vi "JSON-ActorCommand.vi"(6 "Payload":string="Inventory", 8 "error in":errorcluster, 9 "Reply Command":string="ReplyWithAddQuery", 10 "SQL Statement":string, 11 "Table":string="Inventory") -> (0 "error out":errorcluster, 3 "Output JSON Object":string)   [LabVIEW 2013]
uses:
  ftw-dataflow/Actor/src/Utility/FTW-Actor-Configuration.ctl
  ftw-dataflow/Actor/src/FTW-Actor.lvlib
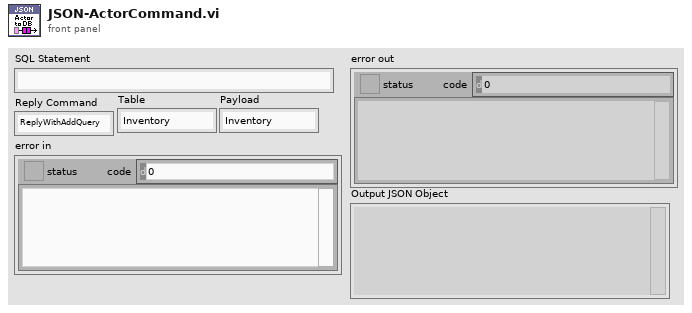
[diagram p1: front panel]
types:
  T1 = typedef "FTW-Actor.lvlib/FTW-Actor-Configuration.ctl" = string
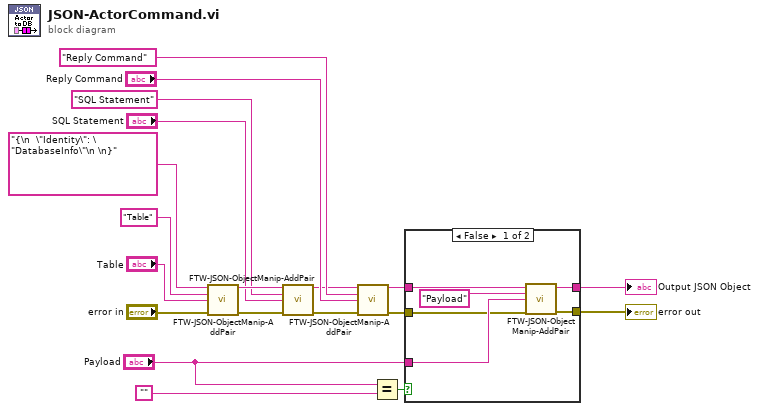
[diagram p0: block diagram]
diagram:
  n1 = call "FTW-JSON-ObjectManip-AddPair.vi"("Input JSON Object"=T1 "{\n  \"Identity\": \"DatabaseInfo\"\n \n}" ("FTW Actor Instance Configuration 2"), "Key"="Table", "Value"="Table", "error in"="error in") -> ("Output JSON Object"=w16:string, "error out"=w9:errorcluster)  [unwired: 10 in]
  n2 = call "FTW-JSON-ObjectManip-AddPair.vi"("Input JSON Object"=w16, "Key"="SQL Statement", "Value"="SQL Statement", "error in"=w9) -> ("Output JSON Object"=w17:string, "error out"=w8:errorcluster)  [unwired: 10 in]
  n3 = call "FTW-JSON-ObjectManip-AddPair.vi"("Input JSON Object"=w17, "Key"="Reply Command", "Value"="Reply Command", "error in"=w8) -> ("Output JSON Object"=w7:string, "error out"=w3:errorcluster)  [unwired: 10 in]
  n4 = Equal?(x="Payload", y="") -> (x = y?=w6:bool)
  n5 = case shown="False" w6 {
    tunnel: w7 -> [w25 w27]
    tunnel: "Payload" -> [w23 _]
    tunnel: w3 -> [w22 w26]
    tunnel: [w21 w26] -> w2
    tunnel: [w20 w27] -> w1
    frame False {
      n6 = call "FTW-JSON-ObjectManip-AddPair.vi"("Input JSON Object"=w25, "Key"="Payload", "Value"=w23, "error in"=w22) -> ("Output JSON Object"=w20:string, "error out"=w21:errorcluster)  [unwired: 10 in]
    }
    frame True {
    }
  }
  "error out" <- w2
  "Output JSON Object" <- w1
